vi "fgv_time-check.vi"(7 "cmd":T1, 8 "error in (no error)":errorcluster) -> (0 "error out":errorcluster, 3 "time check 2":T2)   [LabVIEW 2019]
uses:
  time-check.ctl
  cmd_timecheck.ctl
  SubVIs/common/_ctrl/system-status.ctl
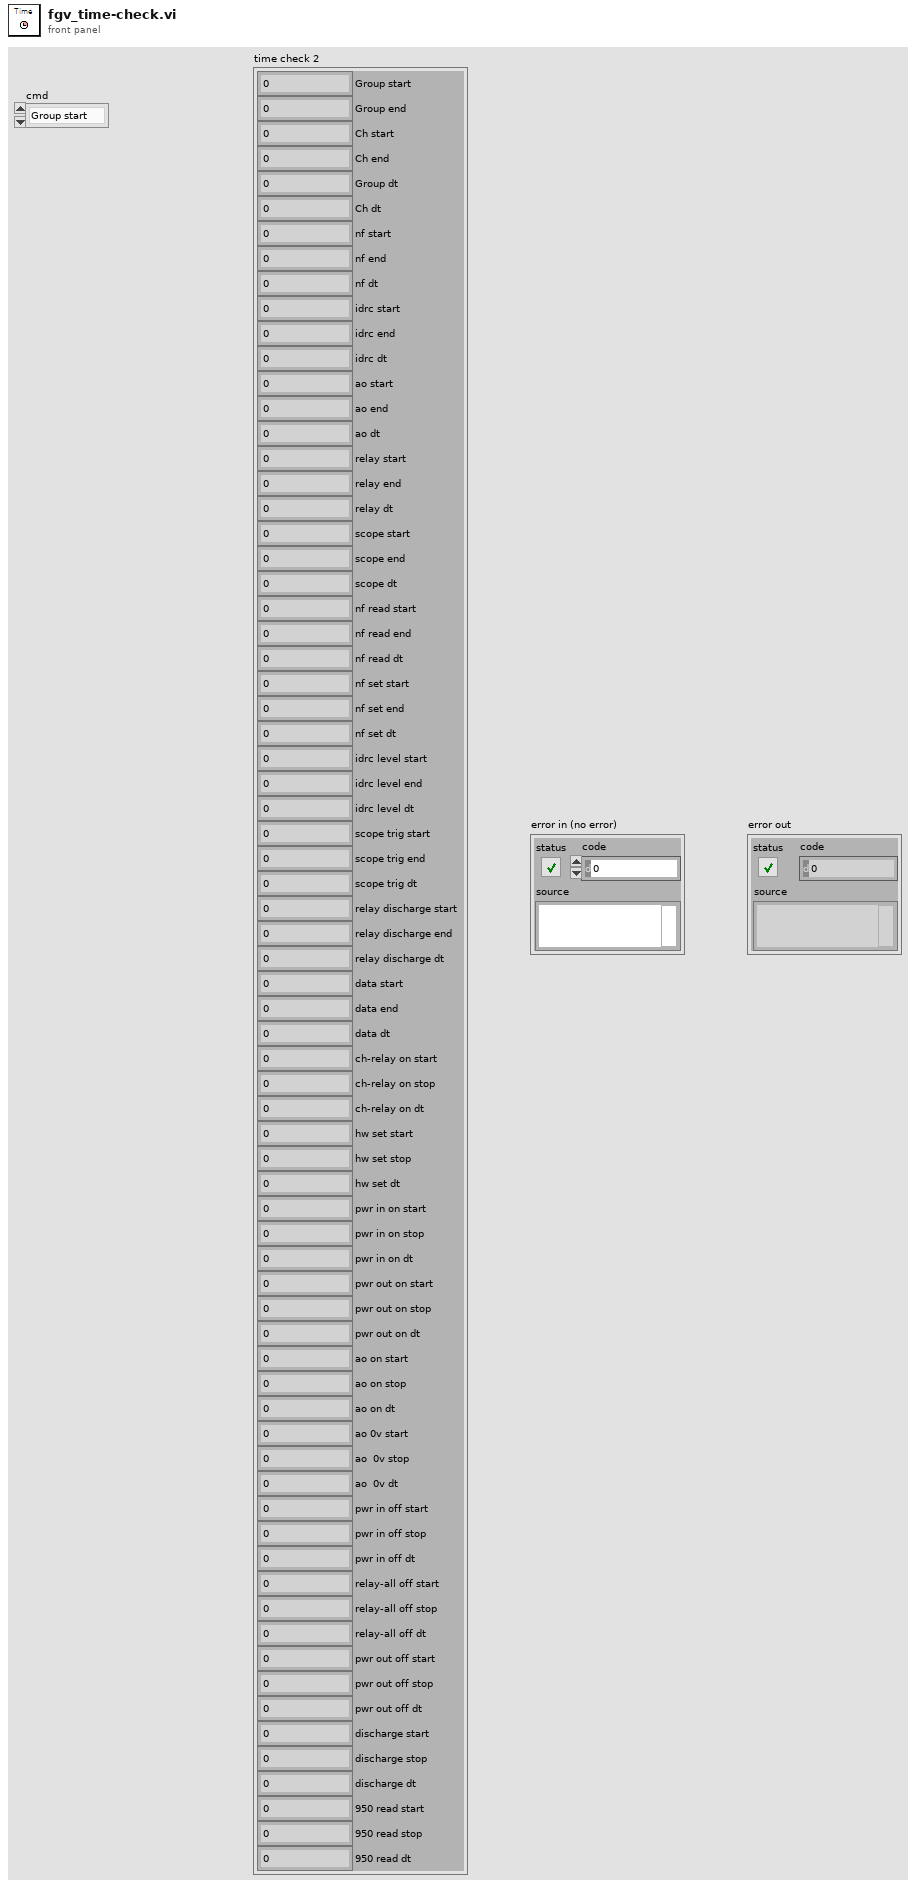
[diagram p1: front panel]
types:
  T1 = typedef "cmd_timecheck.ctl" = enum16{"Group start", "Group end", "Grout dt", "Ch start", "Ch end", "Ch dt", "init", "NF start", "NF stop", "idrc start", "idrc stop", "scope start", "scope stop", "ao start", "ao stop", "relay start", "relay stop", "NF read start", "NF read stop", "NF set start", "NF set stop", "idrc level start", "idrc level stop", "scope trig start", "scope trig stop", "relay dischar star", "relay dischar stop", "data process start", "data process stop", "ch-relay on start", "ch-relay on stop", "hw set start", "hw set stop", "pwr-in on start", "pwr-in on stop", "pwr-out on start", "pwr-out on stop", "ao on start", "ao on stop", "ao 0v start", "ao 0v stop", "pwr-in off start", "pwr-in off stop", "relay-all off start", "relay-all off stop", "pwr-out off start", "pwr-out off stop", "discharge start", "discharge stop", "950 read start", "950 read stop"}
  T2 = typedef "time-check.ctl" = cluster{"Group start":u32, "Group end":u32, "Ch start":u32, "Ch end":u32, "Group dt":dbl, "Ch dt":dbl, "nf start":u32, "nf end":u32, "nf dt":dbl, "idrc start":u32, "idrc end":u32, "idrc dt":dbl, "ao start":u32, "ao end":u32, "ao dt":dbl, "relay start":u32, "relay end":u32, "relay dt":dbl, "scope start":u32, "scope end":u32, "scope dt":dbl, "nf read start":u32, "nf read end":u32, "nf read dt":dbl, "nf set start":u32, "nf set end":u32, "nf set dt":dbl, "idrc level start":u32, "idrc level end":u32, "idrc level dt":dbl, "scope trig start":u32, "scope trig end":u32, "scope trig dt":dbl, "relay discharge start":u32, "relay discharge end":u32, "relay discharge dt ":dbl, "data start":u32, "data end":u32, "data dt":dbl, "ch-relay on start":u32, "ch-relay on stop":u32, "ch-relay on dt":dbl, "hw set start":u32, "hw set stop":u32, "hw set dt":dbl, "pwr in on start":u32, "pwr in on stop":u32, "pwr in on dt":dbl, "pwr out on start":u32, "pwr out on stop":u32, "pwr out on dt":dbl, "ao on start":u32, "ao on stop":u32, "ao on dt":dbl, "ao 0v start":u32, "ao  0v stop":u32, "ao  0v dt":dbl, "pwr in off start":u32, "pwr in off stop":u32, "pwr in off dt":dbl, "relay-all off start":u32, "relay-all off stop":u32, "relay-all off dt":dbl, "pwr out off start":u32, "pwr out off stop":u32, "pwr out off dt":dbl, "discharge start":u32, "discharge stop":u32, "discharge dt":dbl, "950 read start":u32, "950 read stop":u32, "950 read dt":dbl}
  T3 = typedef "system-status.ctl" = enum16{"Initial", "Update", "Clear", "Read"}
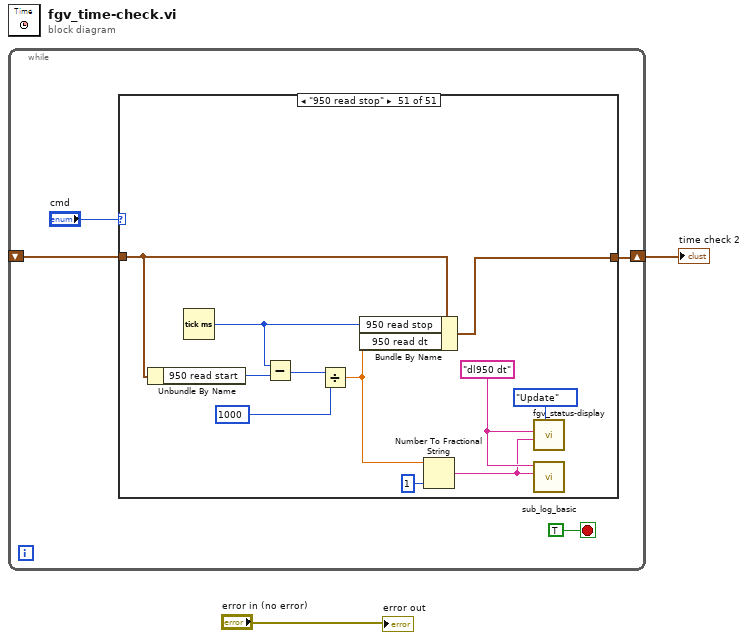
[diagram p0: block diagram]
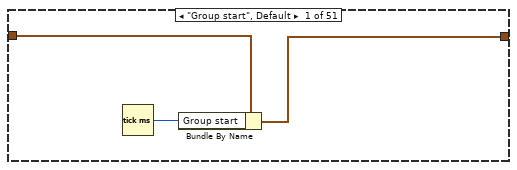
[diagram p2: hidden frame]
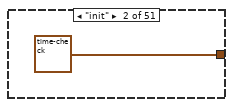
[diagram p3: hidden frame]
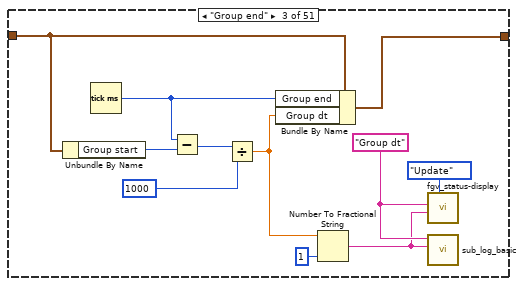
[diagram p4: hidden frame]
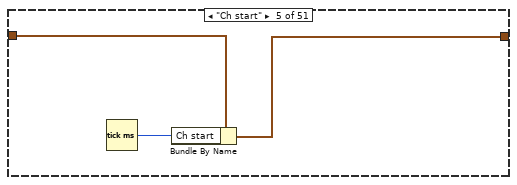
[diagram p6: hidden frame]
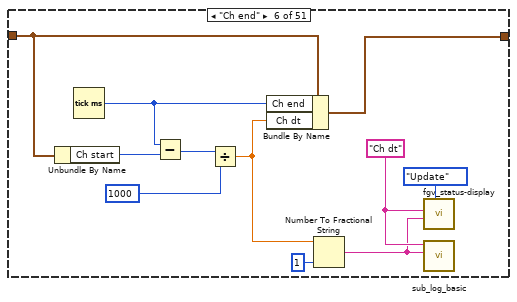
[diagram p7: hidden frame]
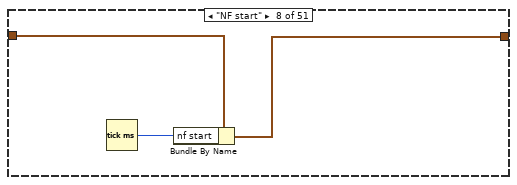
[diagram p9: hidden frame]
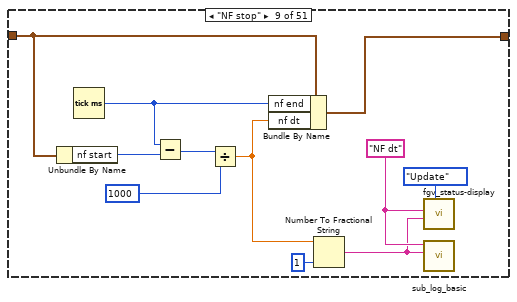
[diagram p10: hidden frame]
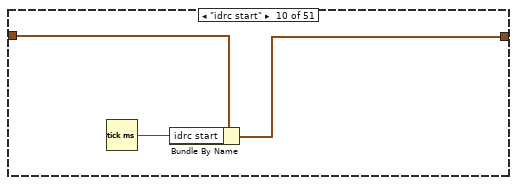
[diagram p11: hidden frame]
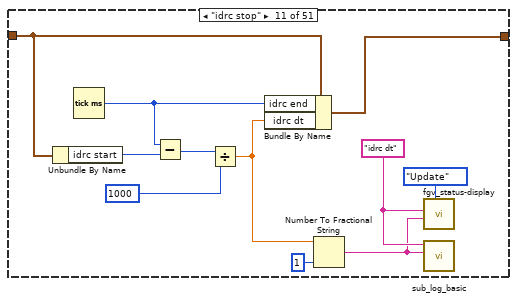
[diagram p12: hidden frame]
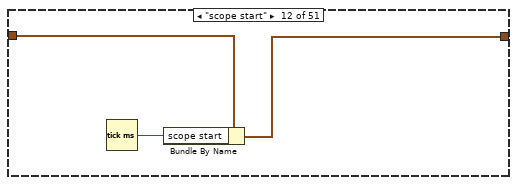
[diagram p13: hidden frame]
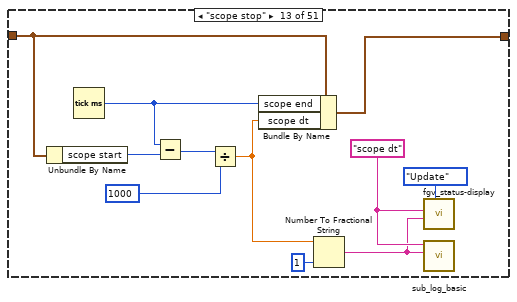
[diagram p14: hidden frame]
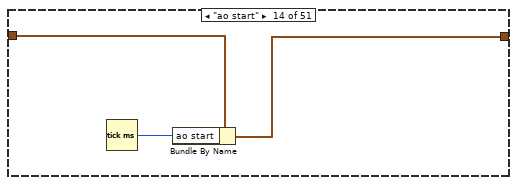
[diagram p15: hidden frame]
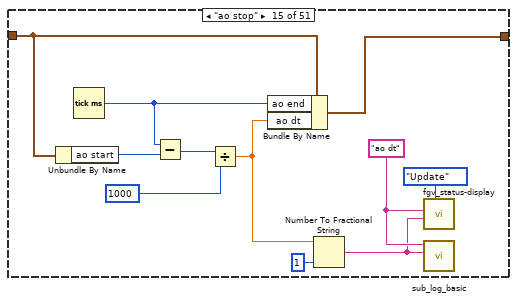
[diagram p16: hidden frame]
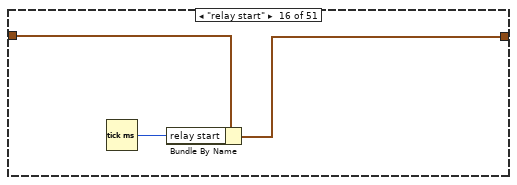
[diagram p17: hidden frame]
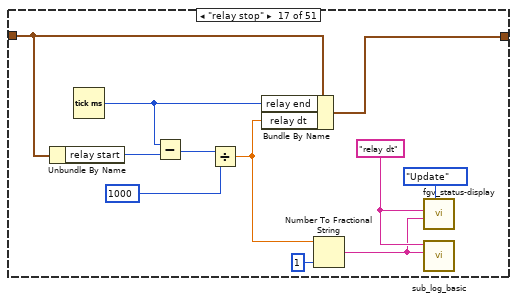
[diagram p18: hidden frame]
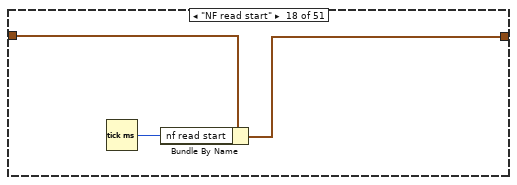
[diagram p19: hidden frame]
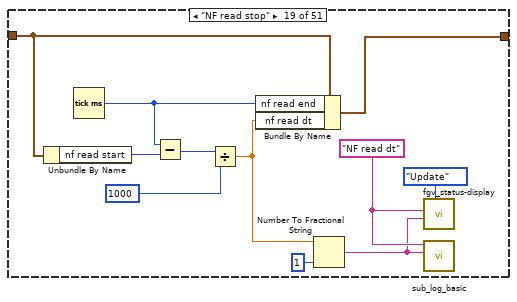
[diagram p20: hidden frame]
diagram:
  n1 = while {
    shift-right: [w5] -> w2
    shift-left: _ -> [w4]
    stop <- TRUE stop-if-true
    n2 = case shown="\"950 read stop\"" "cmd" {
      tunnel: [w8 T2 {"Group start"=0, "Group end"=0, "Ch start"=0, "Ch end"=0, "Group dt"=0.0, "Ch dt"=0.0, "nf start"=0, "nf end"=0, "nf dt"=0.0, "idrc start"=0, "idrc end"=0, "idrc dt"=0.0, "ao start"=0, "ao end"=0, "ao dt"=0.0, "relay start"=0, "relay end"=0, "relay dt"=0.0, "scope start"=0, "scope end"=0, "scope dt"=0.0, "nf read start"=0, "nf read end"=0, "nf read dt"=0.0, "nf set start"=0, "nf set end"=0, "nf set dt"=0.0, "idrc level start"=0, "idrc level end"=0, "idrc level dt"=0.0, "scope trig start"=0, "scope trig end"=0, "scope trig dt"=0.0, "relay discharge start"=0, "relay discharge end"=0, "relay discharge dt "=0.0, "data start"=0, "data end"=0, "data dt"=0.0, "ch-relay on start"=0, "ch-relay on stop"=0, "ch-relay on dt"=0.0, "hw set start"=0, "hw set stop"=0, "hw set dt"=0.0, "pwr in on start"=0, "pwr in on stop"=0, "pwr in on dt"=0.0, "pwr out on start"=0, "pwr out on stop"=0, "pwr out on dt"=0.0, "ao on start"=0, "ao on stop"=0, "ao on dt"=0.0, "ao 0v start"=0, "ao  0v stop"=0, "ao  0v dt"=0.0, "pwr in off start"=0, "pwr in off stop"=0, "pwr in off dt"=0.0, "relay-all off start"=0, "relay-all off stop"=0, "relay-all off dt"=0.0, "pwr out off start"=0, "pwr out off stop"=0, "pwr out off dt"=0.0, "discharge start"=0, "discharge stop"=0, "discharge dt"=0.0, "950 read start"=0, "950 read stop"=0, "950 read dt"=0.0} ("time check") w21 w22 w23 w32 w37 w38 w47 w52 w61 w66 w75 w80 w89 w94 w103 w108 w117 w122 w131 w136 w145 w150 w159 w164 w173 w178 w187 w192 w201 w206 w215 w220 w229 w234 w243 w248 w257 w262 w271 w276 w285 w290 w299 w304 w313 w318 w327 w332 w341] -> w5
      tunnel: w4 -> [w9 _ w20 w22 w24 w31 w37 w39 w46 w53 w60 w67 w74 w81 w88 w95 w102 w109 w116 w123 w130 w137 w144 w151 w158 w165 w172 w179 w186 w193 w200 w207 w214 w221 w228 w235 w242 w249 w256 w263 w270 w277 w284 w291 w298 w305 w312 w319 w326 w333 w340]
      frame "Group start", Default {
        n3 = Tick Count (ms)() -> (millisecond timer value=w7:u32)
        n4 = Bundle By Name(cluster=w9, "Group start"=w7) -> (w8:T2)
      }
      frame "init" {
      }
      frame "Group end" {
        w14 = "Group dt" ("title")
        n5 = Unbundle By Name(w20) -> ("Group start"=w18:u32)
        n6 = Tick Count (ms)() -> (millisecond timer value=w19:u32)
        n7 = Subtract(x=w19, y=w18) -> (x-y=w17:u32)
        n8 = Divide(x=w17, y=u32 1000) -> (x/y=w12:dbl)
        n9 = Bundle By Name(cluster=w20, "Group end"=w19, "Group dt"=w12) -> (w21:T2)
        n10 = Number To Fractional String(number=w12, precision (6)=i16 1) -> (F-format string=w13:string)  [unwired: 2 in]
        n11 = call "fgv_status-display.vi"("Mode"=system-status."Update", "detail"=w13, "title"=w14) -> ()  [unwired: 8 in, 1 out]
        n12 = call "sub_log_basic.vi"("desc"=w13, "Title"=w14) -> ()  [unwired: 9 in, 1 out]
      }
      frame "Grout dt" {
      }
      frame "Ch start" {
        n13 = Tick Count (ms)() -> (millisecond timer value=w25:u32)
        n14 = Bundle By Name(cluster=w24, "Ch start"=w25) -> (w23:T2)
      }
      frame "Ch end" {
        w29 = "Ch dt" ("title")
        n15 = Unbundle By Name(w31) -> ("Ch start"=w35:u32)
        n16 = Tick Count (ms)() -> (millisecond timer value=w36:u32)
        n17 = Subtract(x=w36, y=w35) -> (x-y=w34:u32)
        n18 = Divide(x=w34, y=u32 1000) -> (x/y=w28:dbl)
        n19 = Bundle By Name(cluster=w31, "Ch end"=w36, "Ch dt"=w28) -> (w32:T2)
        n20 = Number To Fractional String(number=w28, precision (6)=i16 1) -> (F-format string=w27:string)  [unwired: 2 in]
        n21 = call "fgv_status-display.vi"("Mode"=system-status."Update", "detail"=w27, "title"=w29) -> ()  [unwired: 8 in, 1 out]
        n22 = call "sub_log_basic.vi"("desc"=w27, "Title"=w29) -> ()  [unwired: 9 in, 1 out]
      }
      frame "Ch dt" {
      }
      frame "NF start" {
        n23 = Tick Count (ms)() -> (millisecond timer value=w40:u32)
        n24 = Bundle By Name(cluster=w39, "nf start"=w40) -> (w38:T2)
      }
      frame "NF stop" {
        w44 = "NF dt" ("title")
        n25 = Unbundle By Name(w46) -> ("nf start"=w50:u32)
        n26 = Tick Count (ms)() -> (millisecond timer value=w51:u32)
        n27 = Subtract(x=w51, y=w50) -> (x-y=w49:u32)
        n28 = Divide(x=w49, y=u32 1000) -> (x/y=w43:dbl)
        n29 = Bundle By Name(cluster=w46, "nf end"=w51, "nf dt"=w43) -> (w47:T2)
        n30 = Number To Fractional String(number=w43, precision (6)=i16 1) -> (F-format string=w42:string)  [unwired: 2 in]
        n31 = call "fgv_status-display.vi"("Mode"=system-status."Update", "detail"=w42, "title"=w44) -> ()  [unwired: 8 in, 1 out]
        n32 = call "sub_log_basic.vi"("desc"=w42, "Title"=w44) -> ()  [unwired: 9 in, 1 out]
      }
      frame "idrc start" {
        n33 = Tick Count (ms)() -> (millisecond timer value=w54:u32)
        n34 = Bundle By Name(cluster=w53, "idrc start"=w54) -> (w52:T2)
      }
      frame "idrc stop" {
        w58 = "idrc dt" ("title")
        n35 = Unbundle By Name(w60) -> ("idrc start"=w64:u32)
        n36 = Tick Count (ms)() -> (millisecond timer value=w65:u32)
        n37 = Subtract(x=w65, y=w64) -> (x-y=w63:u32)
        n38 = Divide(x=w63, y=u32 1000) -> (x/y=w57:dbl)
        n39 = Bundle By Name(cluster=w60, "idrc end"=w65, "idrc dt"=w57) -> (w61:T2)
        n40 = Number To Fractional String(number=w57, precision (6)=i16 1) -> (F-format string=w56:string)  [unwired: 2 in]
        n41 = call "fgv_status-display.vi"("Mode"=system-status."Update", "detail"=w56, "title"=w58) -> ()  [unwired: 8 in, 1 out]
        n42 = call "sub_log_basic.vi"("desc"=w56, "Title"=w58) -> ()  [unwired: 9 in, 1 out]
      }
      frame "scope start" {
        n43 = Tick Count (ms)() -> (millisecond timer value=w68:u32)
        n44 = Bundle By Name(cluster=w67, "scope start"=w68) -> (w66:T2)
      }
      frame "scope stop" {
        w72 = "scope dt" ("title")
        n45 = Unbundle By Name(w74) -> ("scope start"=w78:u32)
        n46 = Tick Count (ms)() -> (millisecond timer value=w79:u32)
        n47 = Subtract(x=w79, y=w78) -> (x-y=w77:u32)
        n48 = Divide(x=w77, y=u32 1000) -> (x/y=w71:dbl)
        n49 = Bundle By Name(cluster=w74, "scope end"=w79, "scope dt"=w71) -> (w75:T2)
        n50 = Number To Fractional String(number=w71, precision (6)=i16 1) -> (F-format string=w70:string)  [unwired: 2 in]
        n51 = call "fgv_status-display.vi"("Mode"=system-status."Update", "detail"=w70, "title"=w72) -> ()  [unwired: 8 in, 1 out]
        n52 = call "sub_log_basic.vi"("desc"=w70, "Title"=w72) -> ()  [unwired: 9 in, 1 out]
      }
      frame "ao start" {
        n53 = Tick Count (ms)() -> (millisecond timer value=w82:u32)
        n54 = Bundle By Name(cluster=w81, "ao start"=w82) -> (w80:T2)
      }
      frame "ao stop" {
        w86 = "ao dt" ("title")
        n55 = Unbundle By Name(w88) -> ("ao start"=w92:u32)
        n56 = Tick Count (ms)() -> (millisecond timer value=w93:u32)
        n57 = Subtract(x=w93, y=w92) -> (x-y=w91:u32)
        n58 = Divide(x=w91, y=u32 1000) -> (x/y=w85:dbl)
        n59 = Bundle By Name(cluster=w88, "ao end"=w93, "ao dt"=w85) -> (w89:T2)
        n60 = Number To Fractional String(number=w85, precision (6)=i16 1) -> (F-format string=w84:string)  [unwired: 2 in]
        n61 = call "fgv_status-display.vi"("Mode"=system-status."Update", "detail"=w84, "title"=w86) -> ()  [unwired: 8 in, 1 out]
        n62 = call "sub_log_basic.vi"("desc"=w84, "Title"=w86) -> ()  [unwired: 9 in, 1 out]
      }
      frame "relay start" {
        n63 = Tick Count (ms)() -> (millisecond timer value=w96:u32)
        n64 = Bundle By Name(cluster=w95, "relay start"=w96) -> (w94:T2)
      }
      frame "relay stop" {
        w100 = "relay dt" ("title")
        n65 = Unbundle By Name(w102) -> ("relay start"=w106:u32)
        n66 = Tick Count (ms)() -> (millisecond timer value=w107:u32)
        n67 = Subtract(x=w107, y=w106) -> (x-y=w105:u32)
        n68 = Divide(x=w105, y=u32 1000) -> (x/y=w99:dbl)
        n69 = Bundle By Name(cluster=w102, "relay end"=w107, "relay dt"=w99) -> (w103:T2)
        n70 = Number To Fractional String(number=w99, precision (6)=i16 1) -> (F-format string=w98:string)  [unwired: 2 in]
        n71 = call "fgv_status-display.vi"("Mode"=system-status."Update", "detail"=w98, "title"=w100) -> ()  [unwired: 8 in, 1 out]
        n72 = call "sub_log_basic.vi"("desc"=w98, "Title"=w100) -> ()  [unwired: 9 in, 1 out]
      }
      frame "NF read start" {
        n73 = Tick Count (ms)() -> (millisecond timer value=w110:u32)
        n74 = Bundle By Name(cluster=w109, "nf read start"=w110) -> (w108:T2)
      }
      frame "NF read stop" {
        w114 = "NF read dt" ("title")
        n75 = Unbundle By Name(w116) -> ("nf read start"=w120:u32)
        n76 = Tick Count (ms)() -> (millisecond timer value=w121:u32)
        n77 = Subtract(x=w121, y=w120) -> (x-y=w119:u32)
        n78 = Divide(x=w119, y=u32 1000) -> (x/y=w113:dbl)
        n79 = Bundle By Name(cluster=w116, "nf read end"=w121, "nf read dt"=w113) -> (w117:T2)
        n80 = Number To Fractional String(number=w113, precision (6)=i16 1) -> (F-format string=w112:string)  [unwired: 2 in]
        n81 = call "fgv_status-display.vi"("Mode"=system-status."Update", "detail"=w112, "title"=w114) -> ()  [unwired: 8 in, 1 out]
        n82 = call "sub_log_basic.vi"("desc"=w112, "Title"=w114) -> ()  [unwired: 9 in, 1 out]
      }
      frame "NF set start" {
        n83 = Tick Count (ms)() -> (millisecond timer value=w124:u32)
        n84 = Bundle By Name(cluster=w123, "nf set start"=w124) -> (w122:T2)
      }
      frame "NF set stop" {
        w128 = "NF set dt" ("title")
        n85 = Unbundle By Name(w130) -> ("nf set start"=w134:u32)
        n86 = Tick Count (ms)() -> (millisecond timer value=w135:u32)
        n87 = Subtract(x=w135, y=w134) -> (x-y=w133:u32)
        n88 = Divide(x=w133, y=u32 1000) -> (x/y=w127:dbl)
        n89 = Bundle By Name(cluster=w130, "nf set end"=w135, "nf set dt"=w127) -> (w131:T2)
        n90 = Number To Fractional String(number=w127, precision (6)=i16 1) -> (F-format string=w126:string)  [unwired: 2 in]
        n91 = call "fgv_status-display.vi"("Mode"=system-status."Update", "detail"=w126, "title"=w128) -> ()  [unwired: 8 in, 1 out]
        n92 = call "sub_log_basic.vi"("desc"=w126, "Title"=w128) -> ()  [unwired: 9 in, 1 out]
      }
      frame "idrc level start" {
        n93 = Tick Count (ms)() -> (millisecond timer value=w138:u32)
        n94 = Bundle By Name(cluster=w137, "idrc level start"=w138) -> (w136:T2)
      }
      frame "idrc level stop" {
        w142 = "idrc level dt" ("title")
        n95 = Unbundle By Name(w144) -> ("idrc level start"=w148:u32)
        n96 = Tick Count (ms)() -> (millisecond timer value=w149:u32)
        n97 = Subtract(x=w149, y=w148) -> (x-y=w147:u32)
        n98 = Divide(x=w147, y=u32 1000) -> (x/y=w141:dbl)
        n99 = Bundle By Name(cluster=w144, "idrc level end"=w149, "idrc level dt"=w141) -> (w145:T2)
        n100 = Number To Fractional String(number=w141, precision (6)=i16 1) -> (F-format string=w140:string)  [unwired: 2 in]
        n101 = call "fgv_status-display.vi"("Mode"=system-status."Update", "detail"=w140, "title"=w142) -> ()  [unwired: 8 in, 1 out]
        n102 = call "sub_log_basic.vi"("desc"=w140, "Title"=w142) -> ()  [unwired: 9 in, 1 out]
      }
      frame "scope trig start" {
        n103 = Tick Count (ms)() -> (millisecond timer value=w152:u32)
        n104 = Bundle By Name(cluster=w151, "scope trig start"=w152) -> (w150:T2)
      }
      frame "scope trig stop" {
        w156 = "scope trig start dt" ("title")
        n105 = Unbundle By Name(w158) -> ("scope trig start"=w162:u32)
        n106 = Tick Count (ms)() -> (millisecond timer value=w163:u32)
        n107 = Subtract(x=w163, y=w162) -> (x-y=w161:u32)
        n108 = Divide(x=w161, y=u32 1000) -> (x/y=w155:dbl)
        n109 = Bundle By Name(cluster=w158, "scope trig end"=w163, "scope trig dt"=w155) -> (w159:T2)
        n110 = Number To Fractional String(number=w155, precision (6)=i16 1) -> (F-format string=w154:string)  [unwired: 2 in]
        n111 = call "fgv_status-display.vi"("Mode"=system-status."Update", "detail"=w154, "title"=w156) -> ()  [unwired: 8 in, 1 out]
        n112 = call "sub_log_basic.vi"("desc"=w154, "Title"=w156) -> ()  [unwired: 9 in, 1 out]
      }
      frame "relay dischar star" {
        n113 = Tick Count (ms)() -> (millisecond timer value=w166:u32)
        n114 = Bundle By Name(cluster=w165, "relay discharge start"=w166) -> (w164:T2)
      }
      frame "relay dischar stop" {
        w170 = "relay discharge dt" ("title")
        n115 = Unbundle By Name(w172) -> ("relay discharge start"=w176:u32)
        n116 = Tick Count (ms)() -> (millisecond timer value=w177:u32)
        n117 = Subtract(x=w177, y=w176) -> (x-y=w175:u32)
        n118 = Divide(x=w175, y=u32 1000) -> (x/y=w169:dbl)
        n119 = Bundle By Name(cluster=w172, "relay discharge end"=w177, "relay discharge dt"=w169) -> (w173:T2)
        n120 = Number To Fractional String(number=w169, precision (6)=i16 1) -> (F-format string=w168:string)  [unwired: 2 in]
        n121 = call "fgv_status-display.vi"("Mode"=system-status."Update", "detail"=w168, "title"=w170) -> ()  [unwired: 8 in, 1 out]
        n122 = call "sub_log_basic.vi"("desc"=w168, "Title"=w170) -> ()  [unwired: 9 in, 1 out]
      }
      frame "data process start" {
        n123 = Tick Count (ms)() -> (millisecond timer value=w180:u32)
        n124 = Bundle By Name(cluster=w179, "data start"=w180) -> (w178:T2)
      }
      frame "data process stop" {
        w184 = "data process dt" ("title")
        n125 = Unbundle By Name(w186) -> ("data start"=w190:u32)
        n126 = Tick Count (ms)() -> (millisecond timer value=w191:u32)
        n127 = Subtract(x=w191, y=w190) -> (x-y=w189:u32)
        n128 = Divide(x=w189, y=u32 1000) -> (x/y=w183:dbl)
        n129 = Bundle By Name(cluster=w186, "data end"=w191, "data dt"=w183) -> (w187:T2)
        n130 = Number To Fractional String(number=w183, precision (6)=i16 1) -> (F-format string=w182:string)  [unwired: 2 in]
        n131 = call "fgv_status-display.vi"("Mode"=system-status."Update", "detail"=w182, "title"=w184) -> ()  [unwired: 8 in, 1 out]
        n132 = call "sub_log_basic.vi"("desc"=w182, "Title"=w184) -> ()  [unwired: 9 in, 1 out]
      }
      frame "ch-relay on start" {
        n133 = Tick Count (ms)() -> (millisecond timer value=w194:u32)
        n134 = Bundle By Name(cluster=w193, "ch-relay on start"=w194) -> (w192:T2)
      }
      frame "ch-relay on stop" {
        w198 = "ch relay on dt" ("title")
        n135 = Unbundle By Name(w200) -> ("ch-relay on start"=w204:u32)
        n136 = Tick Count (ms)() -> (millisecond timer value=w205:u32)
        n137 = Subtract(x=w205, y=w204) -> (x-y=w203:u32)
        n138 = Divide(x=w203, y=u32 1000) -> (x/y=w197:dbl)
        n139 = Bundle By Name(cluster=w200, "ch-relay on stop"=w205, "ch-relay on dt"=w197) -> (w201:T2)
        n140 = Number To Fractional String(number=w197, precision (6)=i16 1) -> (F-format string=w196:string)  [unwired: 2 in]
        n141 = call "fgv_status-display.vi"("Mode"=system-status."Update", "detail"=w196, "title"=w198) -> ()  [unwired: 8 in, 1 out]
        n142 = call "sub_log_basic.vi"("desc"=w196, "Title"=w198) -> ()  [unwired: 9 in, 1 out]
      }
      frame "hw set start" {
        n143 = Tick Count (ms)() -> (millisecond timer value=w208:u32)
        n144 = Bundle By Name(cluster=w207, "hw set start"=w208) -> (w206:T2)
      }
      frame "hw set stop" {
        w212 = "hw set dt" ("title")
        n145 = Unbundle By Name(w214) -> ("hw set start"=w218:u32)
        n146 = Tick Count (ms)() -> (millisecond timer value=w219:u32)
        n147 = Subtract(x=w219, y=w218) -> (x-y=w217:u32)
        n148 = Divide(x=w217, y=u32 1000) -> (x/y=w211:dbl)
        n149 = Bundle By Name(cluster=w214, "hw set stop"=w219, "hw set dt"=w211) -> (w215:T2)
        n150 = Number To Fractional String(number=w211, precision (6)=i16 1) -> (F-format string=w210:string)  [unwired: 2 in]
        n151 = call "fgv_status-display.vi"("Mode"=system-status."Update", "detail"=w210, "title"=w212) -> ()  [unwired: 8 in, 1 out]
        n152 = call "sub_log_basic.vi"("desc"=w210, "Title"=w212) -> ()  [unwired: 9 in, 1 out]
      }
      frame "pwr-in on start" {
        n153 = Tick Count (ms)() -> (millisecond timer value=w222:u32)
        n154 = Bundle By Name(cluster=w221, "pwr in on start"=w222) -> (w220:T2)
      }
      frame "pwr-in on stop" {
        w226 = "pwr in on dt" ("title")
        n155 = Unbundle By Name(w228) -> ("pwr in on start"=w232:u32)
        n156 = Tick Count (ms)() -> (millisecond timer value=w233:u32)
        n157 = Subtract(x=w233, y=w232) -> (x-y=w231:u32)
        n158 = Divide(x=w231, y=u32 1000) -> (x/y=w225:dbl)
        n159 = Bundle By Name(cluster=w228, "pwr in on stop"=w233, "pwr in on dt"=w225) -> (w229:T2)
        n160 = Number To Fractional String(number=w225, precision (6)=i16 1) -> (F-format string=w224:string)  [unwired: 2 in]
        n161 = call "fgv_status-display.vi"("Mode"=system-status."Update", "detail"=w224, "title"=w226) -> ()  [unwired: 8 in, 1 out]
        n162 = call "sub_log_basic.vi"("desc"=w224, "Title"=w226) -> ()  [unwired: 9 in, 1 out]
      }
      frame "pwr-out on start" {
        n163 = Tick Count (ms)() -> (millisecond timer value=w236:u32)
        n164 = Bundle By Name(cluster=w235, "pwr out on start"=w236) -> (w234:T2)
      }
      frame "pwr-out on stop" {
        w240 = "pwr out on dt" ("title")
        n165 = Unbundle By Name(w242) -> ("pwr out on start"=w246:u32)
        n166 = Tick Count (ms)() -> (millisecond timer value=w247:u32)
        n167 = Subtract(x=w247, y=w246) -> (x-y=w245:u32)
        n168 = Divide(x=w245, y=u32 1000) -> (x/y=w239:dbl)
        n169 = Bundle By Name(cluster=w242, "pwr out on stop"=w247, "pwr out on dt"=w239) -> (w243:T2)
        n170 = Number To Fractional String(number=w239, precision (6)=i16 1) -> (F-format string=w238:string)  [unwired: 2 in]
        n171 = call "fgv_status-display.vi"("Mode"=system-status."Update", "detail"=w238, "title"=w240) -> ()  [unwired: 8 in, 1 out]
        n172 = call "sub_log_basic.vi"("desc"=w238, "Title"=w240) -> ()  [unwired: 9 in, 1 out]
      }
      frame "ao on start" {
        n173 = Tick Count (ms)() -> (millisecond timer value=w250:u32)
        n174 = Bundle By Name(cluster=w249, "ao on start"=w250) -> (w248:T2)
      }
      frame "ao on stop" {
        w254 = "ao on dt" ("title")
        n175 = Unbundle By Name(w256) -> ("ao on start"=w260:u32)
        n176 = Tick Count (ms)() -> (millisecond timer value=w261:u32)
        n177 = Subtract(x=w261, y=w260) -> (x-y=w259:u32)
        n178 = Divide(x=w259, y=u32 1000) -> (x/y=w253:dbl)
        n179 = Bundle By Name(cluster=w256, "ao on stop"=w261, "ao on dt"=w253) -> (w257:T2)
        n180 = Number To Fractional String(number=w253, precision (6)=i16 1) -> (F-format string=w252:string)  [unwired: 2 in]
        n181 = call "fgv_status-display.vi"("Mode"=system-status."Update", "detail"=w252, "title"=w254) -> ()  [unwired: 8 in, 1 out]
        n182 = call "sub_log_basic.vi"("desc"=w252, "Title"=w254) -> ()  [unwired: 9 in, 1 out]
      }
      frame "ao 0v start" {
        n183 = Tick Count (ms)() -> (millisecond timer value=w264:u32)
        n184 = Bundle By Name(cluster=w263, "ao 0v start"=w264) -> (w262:T2)
      }
      frame "ao 0v stop" {
        w268 = "ao 0V dt" ("title")
        n185 = Unbundle By Name(w270) -> ("ao 0v start"=w274:u32)
        n186 = Tick Count (ms)() -> (millisecond timer value=w275:u32)
        n187 = Subtract(x=w275, y=w274) -> (x-y=w273:u32)
        n188 = Divide(x=w273, y=u32 1000) -> (x/y=w267:dbl)
        n189 = Bundle By Name(cluster=w270, "ao  0v stop"=w275, "ao  0v dt"=w267) -> (w271:T2)
        n190 = Number To Fractional String(number=w267, precision (6)=i16 1) -> (F-format string=w266:string)  [unwired: 2 in]
        n191 = call "fgv_status-display.vi"("Mode"=system-status."Update", "detail"=w266, "title"=w268) -> ()  [unwired: 8 in, 1 out]
        n192 = call "sub_log_basic.vi"("desc"=w266, "Title"=w268) -> ()  [unwired: 9 in, 1 out]
      }
      frame "pwr-in off start" {
        n193 = Tick Count (ms)() -> (millisecond timer value=w278:u32)
        n194 = Bundle By Name(cluster=w277, "pwr in off start"=w278) -> (w276:T2)
      }
      frame "pwr-in off stop" {
        w282 = "pwr in off dt" ("title")
        n195 = Unbundle By Name(w284) -> ("pwr in off start"=w288:u32)
        n196 = Tick Count (ms)() -> (millisecond timer value=w289:u32)
        n197 = Subtract(x=w289, y=w288) -> (x-y=w287:u32)
        n198 = Divide(x=w287, y=u32 1000) -> (x/y=w281:dbl)
        n199 = Bundle By Name(cluster=w284, "pwr in off stop"=w289, "pwr in off dt"=w281) -> (w285:T2)
        n200 = Number To Fractional String(number=w281, precision (6)=i16 1) -> (F-format string=w280:string)  [unwired: 2 in]
        n201 = call "fgv_status-display.vi"("Mode"=system-status."Update", "detail"=w280, "title"=w282) -> ()  [unwired: 8 in, 1 out]
        n202 = call "sub_log_basic.vi"("desc"=w280, "Title"=w282) -> ()  [unwired: 9 in, 1 out]
      }
      frame "relay-all off start" {
        n203 = Tick Count (ms)() -> (millisecond timer value=w292:u32)
        n204 = Bundle By Name(cluster=w291, "relay-all off start"=w292) -> (w290:T2)
      }
      frame "relay-all off stop" {
        w296 = "relay all off dt" ("title")
        n205 = Unbundle By Name(w298) -> ("relay-all off start"=w302:u32)
        n206 = Tick Count (ms)() -> (millisecond timer value=w303:u32)
        n207 = Subtract(x=w303, y=w302) -> (x-y=w301:u32)
        n208 = Divide(x=w301, y=u32 1000) -> (x/y=w295:dbl)
        n209 = Bundle By Name(cluster=w298, "relay-all off stop"=w303, "relay-all off dt"=w295) -> (w299:T2)
        n210 = Number To Fractional String(number=w295, precision (6)=i16 1) -> (F-format string=w294:string)  [unwired: 2 in]
        n211 = call "fgv_status-display.vi"("Mode"=system-status."Update", "detail"=w294, "title"=w296) -> ()  [unwired: 8 in, 1 out]
        n212 = call "sub_log_basic.vi"("desc"=w294, "Title"=w296) -> ()  [unwired: 9 in, 1 out]
      }
      frame "pwr-out off start" {
        n213 = Tick Count (ms)() -> (millisecond timer value=w306:u32)
        n214 = Bundle By Name(cluster=w305, "pwr out off start"=w306) -> (w304:T2)
      }
      frame "pwr-out off stop" {
        w310 = "pwr out off dt" ("title")
        n215 = Unbundle By Name(w312) -> ("pwr out off start"=w316:u32)
        n216 = Tick Count (ms)() -> (millisecond timer value=w317:u32)
        n217 = Subtract(x=w317, y=w316) -> (x-y=w315:u32)
        n218 = Divide(x=w315, y=u32 1000) -> (x/y=w309:dbl)
        n219 = Bundle By Name(cluster=w312, "pwr out off stop"=w317, "pwr out off dt"=w309) -> (w313:T2)
        n220 = Number To Fractional String(number=w309, precision (6)=i16 1) -> (F-format string=w308:string)  [unwired: 2 in]
        n221 = call "fgv_status-display.vi"("Mode"=system-status."Update", "detail"=w308, "title"=w310) -> ()  [unwired: 8 in, 1 out]
        n222 = call "sub_log_basic.vi"("desc"=w308, "Title"=w310) -> ()  [unwired: 9 in, 1 out]
      }
      frame "discharge start" {
        n223 = Tick Count (ms)() -> (millisecond timer value=w320:u32)
        n224 = Bundle By Name(cluster=w319, "discharge start"=w320) -> (w318:T2)
      }
      frame "discharge stop" {
        w324 = "discharge dt" ("title")
        n225 = Unbundle By Name(w326) -> ("discharge start"=w330:u32)
        n226 = Tick Count (ms)() -> (millisecond timer value=w331:u32)
        n227 = Subtract(x=w331, y=w330) -> (x-y=w329:u32)
        n228 = Divide(x=w329, y=u32 1000) -> (x/y=w323:dbl)
        n229 = Bundle By Name(cluster=w326, "discharge stop"=w331, "discharge dt"=w323) -> (w327:T2)
        n230 = Number To Fractional String(number=w323, precision (6)=i16 1) -> (F-format string=w322:string)  [unwired: 2 in]
        n231 = call "fgv_status-display.vi"("Mode"=system-status."Update", "detail"=w322, "title"=w324) -> ()  [unwired: 8 in, 1 out]
        n232 = call "sub_log_basic.vi"("desc"=w322, "Title"=w324) -> ()  [unwired: 9 in, 1 out]
      }
      frame "950 read start" {
        n233 = Tick Count (ms)() -> (millisecond timer value=w334:u32)
        n234 = Bundle By Name(cluster=w333, "950 read start"=w334) -> (w332:T2)
      }
      frame "950 read stop" {
        w338 = "dl950 dt" ("title")
        n235 = Unbundle By Name(w340) -> ("950 read start"=w344:u32)
        n236 = Tick Count (ms)() -> (millisecond timer value=w345:u32)
        n237 = Subtract(x=w345, y=w344) -> (x-y=w343:u32)
        n238 = Divide(x=w343, y=u32 1000) -> (x/y=w337:dbl)
        n239 = Bundle By Name(cluster=w340, "950 read stop"=w345, "950 read dt"=w337) -> (w341:T2)
        n240 = Number To Fractional String(number=w337, precision (6)=i16 1) -> (F-format string=w336:string)  [unwired: 2 in]
        n241 = call "fgv_status-display.vi"("Mode"=system-status."Update", "detail"=w336, "title"=w338) -> ()  [unwired: 8 in, 1 out]
        n242 = call "sub_log_basic.vi"("desc"=w336, "Title"=w338) -> ()  [unwired: 9 in, 1 out]
      }
    }
  }
  "time check 2" <- w2
  "error out" <- "error in (no error)"
